vi "Shift_register.vi"() -> ()   [LabVIEW 2018]
panel:
  in  "stop":bool
  out "x-3":dbl
  out "x-2":dbl
  out "x-1":dbl
  out "x":dbl
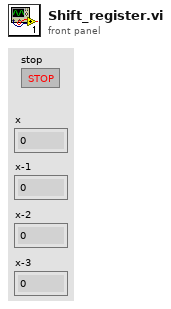
[diagram p1: front panel]
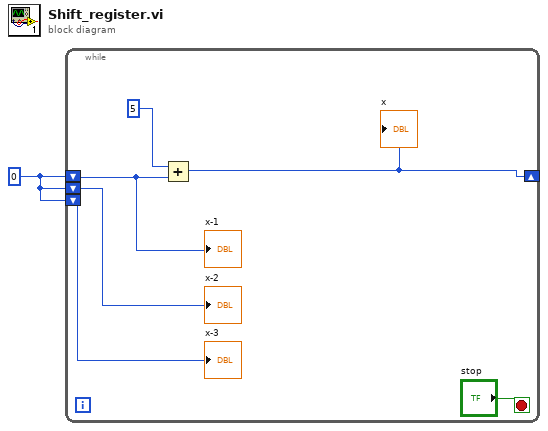
[diagram p0: block diagram]
diagram:
  w1 = 0
  n1 = while {
    shift-right: [w6] -> _
    shift-left: w1 -> [w3]
    shift-left: w1 -> [w4]
    shift-left: w1 -> [w5]
    stop <- "stop" stop-if-true
    n2 = Add(x=5, y=w3) -> (x+y=w6:i32)
    "x" <- w6
    "x-1" <- w3
    "x-2" <- w4
    "x-3" <- w5
  }
